vi "xiC - IMAQ - DetectDeviceType.vi"(8 "error in (no error)":errorcluster, 11 "Attributes In":T1) -> (0 "error out":errorcluster, 3 "Attributes Out":T1)   [LabVIEW 2015]
uses:
  xiCamLib/xiLIB/Typedefs/xiLIB - Device_Type.ctl
  xiCamLib/xiCam/PRM/PRM/PRM_v2.ctl
  C:/GIT/Cameras3.x/Integrations/Labview/xiLib/xiLIB_32bit/xiLIB/xiCamLib/xiLIB/Typedefs/xiLIB - Device_Type.ctl
  xiC - IMAQ - Attributes.ctl
  C:/GIT/Cameras3.x/Integrations/Labview/xiLib/xiLIB_32bit/xiLIB/xiCamLib/API/x86/xiApi.NET.dll
  xiLIB_32bit/xiLIB/xiCamLib/API/x86/xiApi.NET.dll
  xiC - IMAQ - TreeDisplayType.ctl
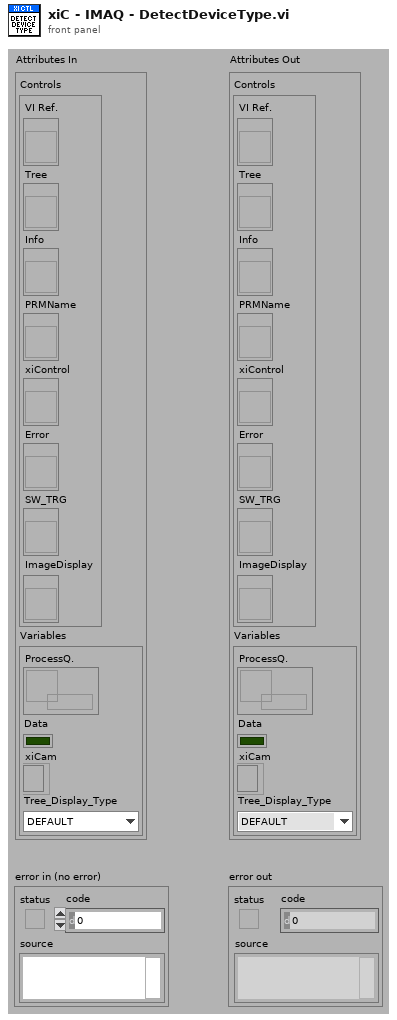
[diagram p1: front panel]
types:
  T1 = typedef "xiC - IMAQ - Attributes.ctl" = cluster{"Controls":cluster{"VI Ref.":refnum<vi>, "Tree":refnum<vi>, "Info":refnum<vi>, "PRMName":refnum<vi>, "xiControl":refnum<vi>, "Error":refnum<vi>, "SW_TRG":refnum<vi>, "ImageDisplay":refnum<vi>}, "Variables":cluster{"ProcessQ.":refnum<queue>, "Data":bool, "xiCam":refnum<k24>, "Tree_Display_Type":T2}}
  T2 = typedef "xiC - IMAQ - TreeDisplayType.ctl" = enum16{"DEFAULT", "HIDE_MAX_MIN"}
  T3 = typedef "xiLIB - Device_Type.ctl" = enum16{"USB2.0", "USB3.0", "CURRERA", "PCIe", "1394"}
  T4 = typedef "PRM_v2.ctl" = enum16{"ACQ_BUFFER_SIZE", "ACQ_FRAME_BURST_COUNT", "ACQ_TIMING_MODE", "ACQ_TRANSPORT_BUFFER_SIZE", "AE_MAX_LIMIT", "AEAG", "AEAG_LEVEL", "API_VERSION", "AG_MAX_LIMIT", "APPLY_CMS", "AUTO_BANDWIDTH_CALCULATION", "AUTO_WB", "AVAILABLE_BANDWIDTH", "AVAILABLE_BANDWIDTH_MAX", "AVAILABLE_BANDWIDTH_MIN", "BPC", "BUFFER_POLICY", "BUFFERS_QUEUE_SIZE", "CC_MATRIX_00", "CC_MATRIX_01", "CC_MATRIX_02", "CC_MATRIX_03", "CC_MATRIX_10", "CC_MATRIX_11", "CC_MATRIX_12", "CC_MATRIX_13", "CC_MATRIX_20", "CC_MATRIX_21", "CC_MATRIX_22", "CC_MATRIX_23", "CC_MATRIX_30", "CC_MATRIX_31", "CC_MATRIX_32", "CC_MATRIX_33", "CHIP_TEMP", "CMS", "COLOR_FILTER_ARRAY", "COOLING", "DEBOUNCE_EN", "DEBOUNCE_POL", "DEBOUNCE_T0", "DEBOUNCE_T1", "DEBUG_LEVEL", "DEFAULT_CC_MATRIX", "DEVICE_INSTANCE_PATH", "DEVICE_MODEL_ID", "DEVICE_NAME", "DEVICE_SN", "DEVICE_TYPE", "DEVICE_USER_ID", "DOWNSAMPLING", "DOWNSAMPLING_MAX", "DOWNSAMPLING_MIN", "DOWNSAMPLING_TYPE", "DRV_VERSION", "EXP_PRIORITY", "EXPOSURE", "EXPOSURE_DIRECT_UPDATE", "EXPOSURE_MAX", "EXPOSURE_MIN", "FFS_FILE_NAME", "FPGA1_VERSION", "FRAMERATE", "FRAMERATE_MAX", "FRAMERATE_MIN", "FREE_FFS_SIZE", "GAIN", "GAIN_DIRECT_UPDATE", "GAIN_MAX", "GAIN_MIN", "GAMMAC", "GAMMAY", "GPI_LEVEL", "GPI_MODE", "GPI_SELECTOR", "GPI_SELECTOR_MAX", "GPI_SELECTOR_MIN", "GPO_MODE", "GPO_SELECTOR", "GPO_SELECTOR_MAX", "GPO_SELECTOR_MIN", "HDR", "HDR_T1", "HDR_T2", "HEIGHT", "HEIGHT_MAX", "HEIGHT_MIN", "HOUSE_TEMP", "IMAGE_DATA_FORMAT", "IMAGE_IS_COLOR", "INPUT_CMS_PROFILE", "IS_COOLED", "IS_DEVICE_EXIST", "KNEEPOINT1", "KNEEPOINT2", "LED_MODE", "LED_SELECTOR", "LED_SELECTOR_MAX", "LED_SELECTOR_MIN", "LIMIT_BANDWIDTH", "LIMIT_BANDWIDTH_MAX", "LIMIT_BANDWIDTH_MIN", "LUT_EN", "LUT_INDEX", "LUT_INDEX_MAX", "LUT_INDEX_MIN", "LUT_VALUE", "LUT_VALUE_MAX", "LUT_VALUE_MIN", "MANUAL_WB", "MCU1_VERSION", "MCU2_VERSION", "OFFSET_X", "OFFSET_X_MAX", "OFFSET_X_MIN", "OFFSET_Y", "OFFSET_Y_MAX", "OFFSET_Y_MIN", "OUTPUT_CMS_PROFILE", "OUTPUT_DATA_BIT_DEPTH", "OUTPUT_DATA_PACKING", "READ_FILE_FFS", "RECENT_FRAME", "SENSOR_DATA_BIT_DEPTH", "SENSOR_MODE", "SENSOR_TAPS", "SHARPNESS", "SHUTTER_TYPE", "TARGET_TEMP", "TRG_DELAY", "TRG_SELECTOR", "TRG_SOFTWARE", "TRG_SOURCE", "USED_FFS_SIZE", "WB_KB", "WB_KG", "WB_KR", "WIDTH", "WIDTH_MAX", "WIDTH_MIN", "WRITE_FILE_FFS", "ACQ_BUFFER_SIZE_UNIT", "ACQ_TRANSPORT_BUFFER_COMMIT", "AEAG_ROI_HEIGHT", "AEAG_ROI_OFFSET_X", "AEAG_ROU_OFFSET_Y", "AEAG_ROI_WIDTH", "API_CONTEXT_LIST", "BINNING_HORIZONTAL", "BINNING_SELECTOR", "BINNING_VERTICAL", "COLUMN_FPN_CORRECTION", "COUNTER_SELECTOR", "COUNTER_VALUE", "DECIMATION_HORIZONTAL", "DECIMATION_SELECTOR", "DECIMATION_VERTICAL", "DEVICE_ID", "DEVICE_LOCATION_PATH", "DEVICE_MANIFEST", "DEVICE_RESET", "DEVICE_SENS_SN", "EXPOSURE_BURST_COUNT", "FFS_ACCESS_KEY", "GAIN_SELECTOR", "HW_REVISION", "IMAGE_BLACK_LEVEL", "IMAGE_DATA_BIT_DEPTH", "IMAGE_DATA_FORMAT_RGB32_ALPHA", "IMAGE_PAYLOAD_SIZE", "LENS_APERTURE_VALUE", "LENS_FEATURE", "LENS_FEATURE_SELECTOR", "LENS_FOCAL_LENGTH", "LENS_FOCUS_DISTANCE", "LENS_FOCUS_MOVE", "LENS_FOCUS_MOVEMENT_VALUE", "LENS_MODE", "OUTPUT_DATA_PACKING_TYPE", "SENSOR_CLOCK_FREQ_HZ", "SENSOR_CLOCK_FREQ_INDEX", "SENSOR_FEATURE_SELECTOR", "SENSOR_FEATURE_VALUE", "SENSOR_OUTPUT_CHANNEL_COUNT", "TRANSPORT_PIXEL_FORMAT", "TS_RST_MODE", "TS_RST_SOURCE"}
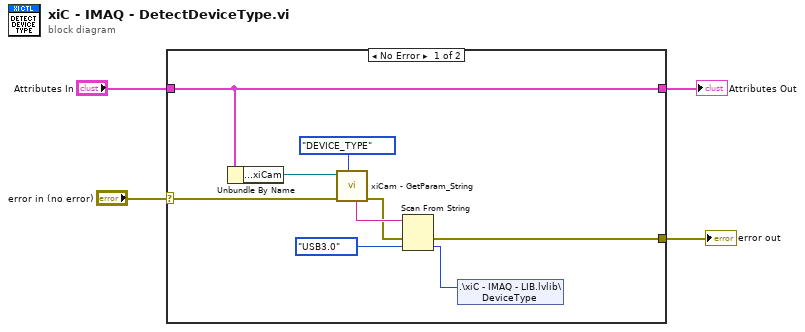
[diagram p0: block diagram]
diagram:
  n1 = case shown="No Error" "error in (no error)" {
    selector: "error in (no error)" -> [w11 w15]
    tunnel: [w6 w15] -> w3
    tunnel: "Attributes In" -> [w12 w14]
    tunnel: [w12 w14] -> w1
    frame No Error {
      n2 = Unbundle By Name(w12) -> ("Variables.xiCam"=w13:refnum<k24>)
      n3 = call "xiCam - GetParam_String.vi"("PRM"=PRM_v2."DEVICE_TYPE", "error in (no error)"=w11, "xiCam In"=w13) -> ("error out"=w7:errorcluster, "String_Value"=w9:string)  [unwired: 6 in, 1 out]
      n4 = Scan From String(input string=w9, error in=w7, default 1=xiLIB_-_Device_Type."USB3.0" ("xiDeviceType")) -> (error out=w6:errorcluster, output 1=w5:T3)  [unwired: 2 in, 2 out]
      n5 = shared-variable ".\\xiC - IMAQ - LIB.lvlib\\DeviceType"(w5) -> ()  [unwired: 1 in, 1 out]
    }
    frame Error {
    }
  }
  "error out" <- w3
  "Attributes Out" <- w1
